vi "Read prev ixon op mode.vi"(8 "error in (no error)":errorcluster, 11 "Sim_Ixon_Ultra in":refnum<class "Sim_Ixon_Ultra.lvclass">) -> (0 "error out":errorcluster, 1 "prev operation mode":T1, 2 "prev ixon op mode":T2={"EM_MODE"=20, "EM_GAIN"=0, "FRAME_TRANSFER"=FALSE}, 3 "Sim_Ixon_Ultra out":refnum<class "Sim_Ixon_Ultra.lvclass">)   [LabVIEW 2018, in "Sim_Ixon_Ultra.lvclass"]
uses:
  Sim_Ixon_Ultra.lvclass
  C:/Users/Denis/Desktop/S4ACS/S4ACS/Simulated_CCD_Camera/Simulated Camera.lvclass
  Sim_Ixon_Ultra.lvclass/Sim_Ixon_Ultra.ctl
  Simulated_CCD_Camera/Simulated Camera.lvclass
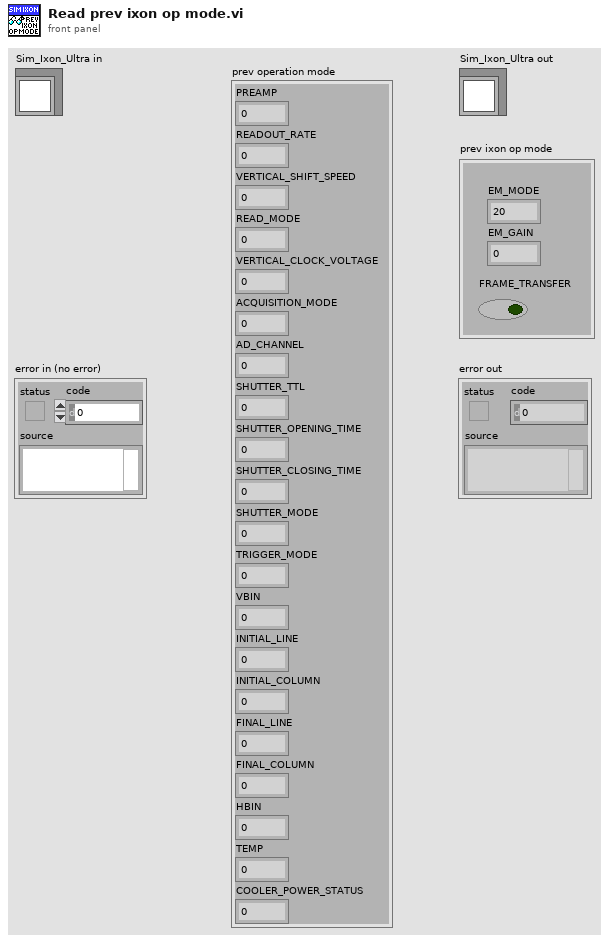
[diagram p1: front panel]
types:
  T1 = cluster{"PREAMP":u16, "READOUT_RATE":u16, "VERTICAL_SHIFT_SPEED":u16, "READ_MODE":u16, "VERTICAL_CLOCK_VOLTAGE":u16, "ACQUISITION_MODE":u16, "AD_CHANNEL":u16, "SHUTTER_TTL":u16, "SHUTTER_OPENING_TIME":u16, "SHUTTER_CLOSING_TIME":u16, "SHUTTER_MODE":u16, "TRIGGER_MODE":u16, "VBIN":u16, "INITIAL_LINE":u16, "INITIAL_COLUMN":u16, "FINAL_LINE":u16, "FINAL_COLUMN":u16, "HBIN":u16, "TEMP":i32, "COOLER_POWER_STATUS":u16}
  T2 = cluster{"EM_MODE":u16, "EM_GAIN":u16, "FRAME_TRANSFER":bool}
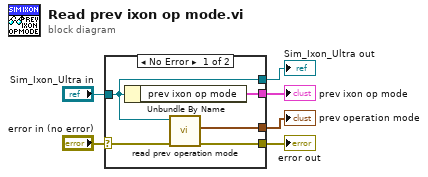
[diagram p0: block diagram]
diagram:
  n1 = case shown="No Error" "error in (no error)" {
    selector: "error in (no error)" -> [w9 w12]
    tunnel: [w8 w12] -> w5
    tunnel: [w10 w13] -> w3
    tunnel: "Sim_Ixon_Ultra in" -> [w10 w13]
    tunnel: [w11 _] -> w2
    tunnel: [w7 _] -> w1
    frame No Error {
      n2 = Unbundle By Name(w10) -> ("prev ixon op mode"=w11:T2)
      n3 = call "read prev operation mode.vi"("error in (no error)"=w9, "Simulated_CCD_Camera in"=w10) -> ("error out"=w8:errorcluster, "prev operation mode"=w7:T1)  [unwired: 7 in, 1 out]
    }
    frame Error {
    }
  }
  "error out" <- w5
  "Sim_Ixon_Ultra out" <- w3
  "prev ixon op mode" <- w2
  "prev operation mode" <- w1
